vi "Controller Open Ethercat Variables.vi"(8 "error in (no error)":errorcluster, 11 "FOFB Configuration":T3={"FOFB Parameters"={"Network"={"FOFB Controller IP"="", "LNLS Control Network IP"="", "LNLS Control Network Power Supplies TCP Port"=0, "LNLS Control Network FOFB Configuration TCP Port"=0, "Data Server TCP Port"=0, "Monitoring Data TCP Port"=0, "Configuration GUI TCP Port"=0, "TCP Listening Timeout"=0}, "Fast Acquisition"={"Acquisition Period"=0, "Data Buffer Size"=0}, "Response Matrix Measurement"={"Step Amplitude"=0.0, "Time Between Steps"=0, "Step Duration"=0, "Number of Averages"=0}, "Correction Algorithm"={"Correction Period"=0, "Reference Orbit Path"=path "", "Response Matrix Path"=path "", "Correction Matrix Path"=path "", "Horizontal Correction Factor"=0.0, "Vertical Correction Factor"=0.0, "Beam Current FOFB Threshold"=0.0, "Decouple H-V"=FALSE}, "Acquisition Network"=[], "Actuation Network"=[]}, "Number of Acquisition Chassis"=0, "Number of Actuation Chassis"=0, "Number of BPM Readings"=0, "BPM Reading Names"=[], "Selected BPM Readings"=[0, 1, 2, 3, 4, 5, 6, 7, 8, 9, 10, 11, 12, 13, 14, 15, 16, 17, 18, 19, 20, 21, 22, 23, 24, 25, 26, 27, 28, 29, 30, 31, 32, 33, 34, 35, 36, 37, 38, 39, 40, 41, 42, 43, 44, 45, 46, 47, 48, 49], "Number of Correctors"=0, "Corrector Names"=[], "Selected Correctors"=[0, 1, 2, 3, 4, 5, 6, 7, 8, 9, 10, 11, 12, 13, 14, 15, 16, 17, 18, 19, 20, 21, 22, 23, 24, 25, 26, 27, 28, 29, 30, 31, 32, 33, 34, 35, 36, 37, 38, 39, 40, 41, 42, 43, 44, 45, 46, 47, 48, 49], "Reference Orbit"=[], "Response Matrix"=[], "Correction Matrix"=[], "Acquisition Chassis Names"=[], "Actuation Chassis Names"=[], "Acquisition Variables"=[], "Actuation Variables"=[], "PS Matrix Mapping"=[], "Inverse PS Matrix Mapping"=[], "Response Matrix Beam Energy (MeV)"=0.0, "PID Parameters"=[], "BPM Planes"=[], "Corrector Planes"=[], "RMM Step Factor"=[]}) -> (0 "error out":errorcluster, 2 "PS Variables":T1, 3 "BPM Variables":T2)   [LabVIEW 2011, in "Controller VIs.lvlib"]
doc: "Open references for all Acquisition and Actuation variables which are used to exchange data between the FOFB Controller and the Acquisition/Actuation chassis via the EtherCAT networks."
uses:
  Controller VIs.lvlib
  Types Definitions/Type FOFB Configuration.ctl
  Types Definitions/Type FOFB Parameters.ctl
  Types Definitions/Type Network Configuration.ctl
  Types Definitions/Type FA Configuration.ctl
  Types Definitions/Type Response Matrix Measurement Configuration.ctl
  Types Definitions/Type Correction Algorithm Configuration.ctl
  Types Definitions/Type Acquisition Network Configuration.ctl
  Types Definitions/Type Actuation Network Configuration.ctl
  Types Definitions/Type PID Parameters.ctl
  Types Definitions/Type BPM Variables.ctl
  Types Definitions/Type PS Variables.ctl
  Type Definitions.lvlib
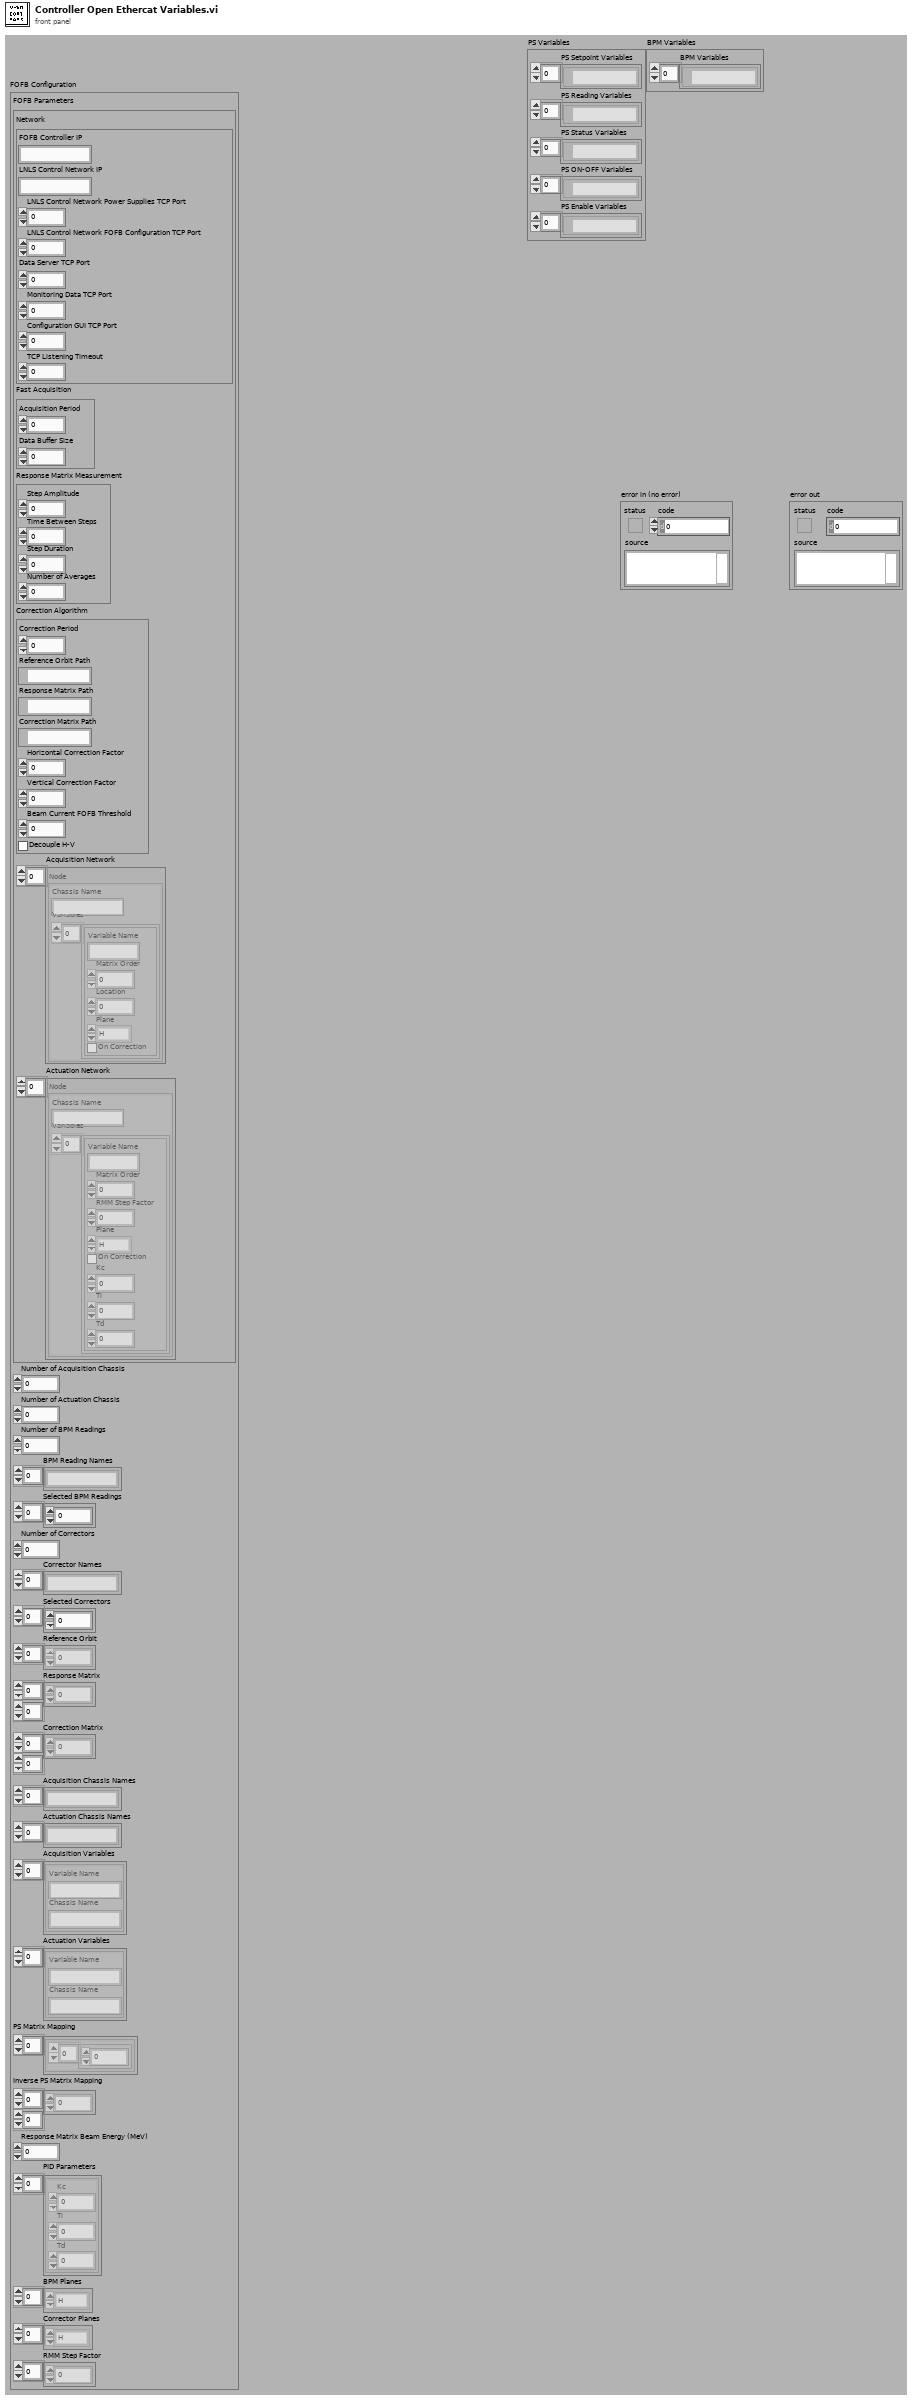
[diagram p1: front panel]
types:
  T1 = typedef "Type Definitions.lvlib/Type PS Variables.ctl" = cluster{"PS Setpoint Variables":refnum<k21>[], "PS Reading Variables":refnum<k21>[], "PS Status Variables":refnum<k21>[], "PS ON-OFF Variables":refnum<k21>[], "PS Enable Variables":refnum<k21>[]}
  T2 = typedef "Type Definitions.lvlib/Type BPM Variables.ctl" = cluster{"BPM Variables":refnum<k21>[]}
  T3 = typedef "Type Definitions.lvlib/Type FOFB Configuration.ctl" = cluster{"FOFB Parameters":T4, "Number of Acquisition Chassis":i32, "Number of Actuation Chassis":i32, "Number of BPM Readings":i32, "BPM Reading Names":string[], "Selected BPM Readings":u32[], "Number of Correctors":i32, "Corrector Names":string[], "Selected Correctors":u32[], "Reference Orbit":dbl[], "Response Matrix":dbl[][], "Correction Matrix":dbl[][], "Acquisition Chassis Names":string[], "Actuation Chassis Names":string[], "Acquisition Variables":cluster{"Variable Name":string, "Chassis Name":string}[], "Actuation Variables":cluster{"Variable Name":string, "Chassis Name":string}[], "PS Matrix Mapping":cluster{u32[]}[], "Inverse PS Matrix Mapping":u32[][], "Response Matrix Beam Energy (MeV)":dbl, "PID Parameters":T11[], "BPM Planes":enum8{"H", "V"}[], "Corrector Planes":enum8{"H", "V"}[], "RMM Step Factor":dbl[]}
  T4 = typedef "Type Definitions.lvlib/Type FOFB Parameters.ctl" = cluster{"Network":T5, "Fast Acquisition":T6, "Response Matrix Measurement":T7, "Correction Algorithm":T8, "Acquisition Network":T9, "Actuation Network":T10}
  T5 = typedef "Type Definitions.lvlib/Type Network Configuration.ctl" = cluster{"FOFB Controller IP":string, "LNLS Control Network IP":string, "LNLS Control Network Power Supplies TCP Port":u16, "LNLS Control Network FOFB Configuration TCP Port":u16, "Data Server TCP Port":u16, "Monitoring Data TCP Port":u16, "Configuration GUI TCP Port":u16, "TCP Listening Timeout":i32}
  T6 = typedef "Type Definitions.lvlib/Type FA Configuration.ctl" = cluster{"Acquisition Period":u32, "Data Buffer Size":u32}
  T7 = typedef "Type Definitions.lvlib/Type Response Matrix Measurement Configuration.ctl" = cluster{"Step Amplitude":dbl, "Time Between Steps":u32, "Step Duration":u32, "Number of Averages":u32}
  T8 = typedef "Type Definitions.lvlib/Type Correction Algorithm Configuration.ctl" = cluster{"Correction Period":u32, "Reference Orbit Path":path, "Response Matrix Path":path, "Correction Matrix Path":path, "Horizontal Correction Factor":dbl, "Vertical Correction Factor":dbl, "Beam Current FOFB Threshold":dbl, "Decouple H-V":bool}
  T9 = typedef "Type Definitions.lvlib/Type Acquisition Network Configuration.ctl" = cluster{"Chassis Name":string, "Variables":cluster{"Variable Name":string, "Matrix Order":u32, "Location":dbl, "Plane":enum8{"H", "V"}, "On Correction":bool}[]}[]
  T10 = typedef "Type Definitions.lvlib/Type Actuation Network Configuration.ctl" = cluster{"Chassis Name":string, "Variables":cluster{"Variable Name":string, "Matrix Order":u32, "RMM Step Factor":dbl, "Plane":enum8{"H", "V"}, "On Correction":bool, "Kc":dbl, "Ti":dbl, "Td":dbl}[]}[]
  T11 = typedef "Type Definitions.lvlib/Type PID Parameters.ctl" = cluster{"Kc":fxp<+/-,16,8>, "Ti":fxp<+/-,16,8>, "Td":fxp<+/-,16,8>}
  T12 = cluster{"Variable Name":string, "Chassis Name":string}[]
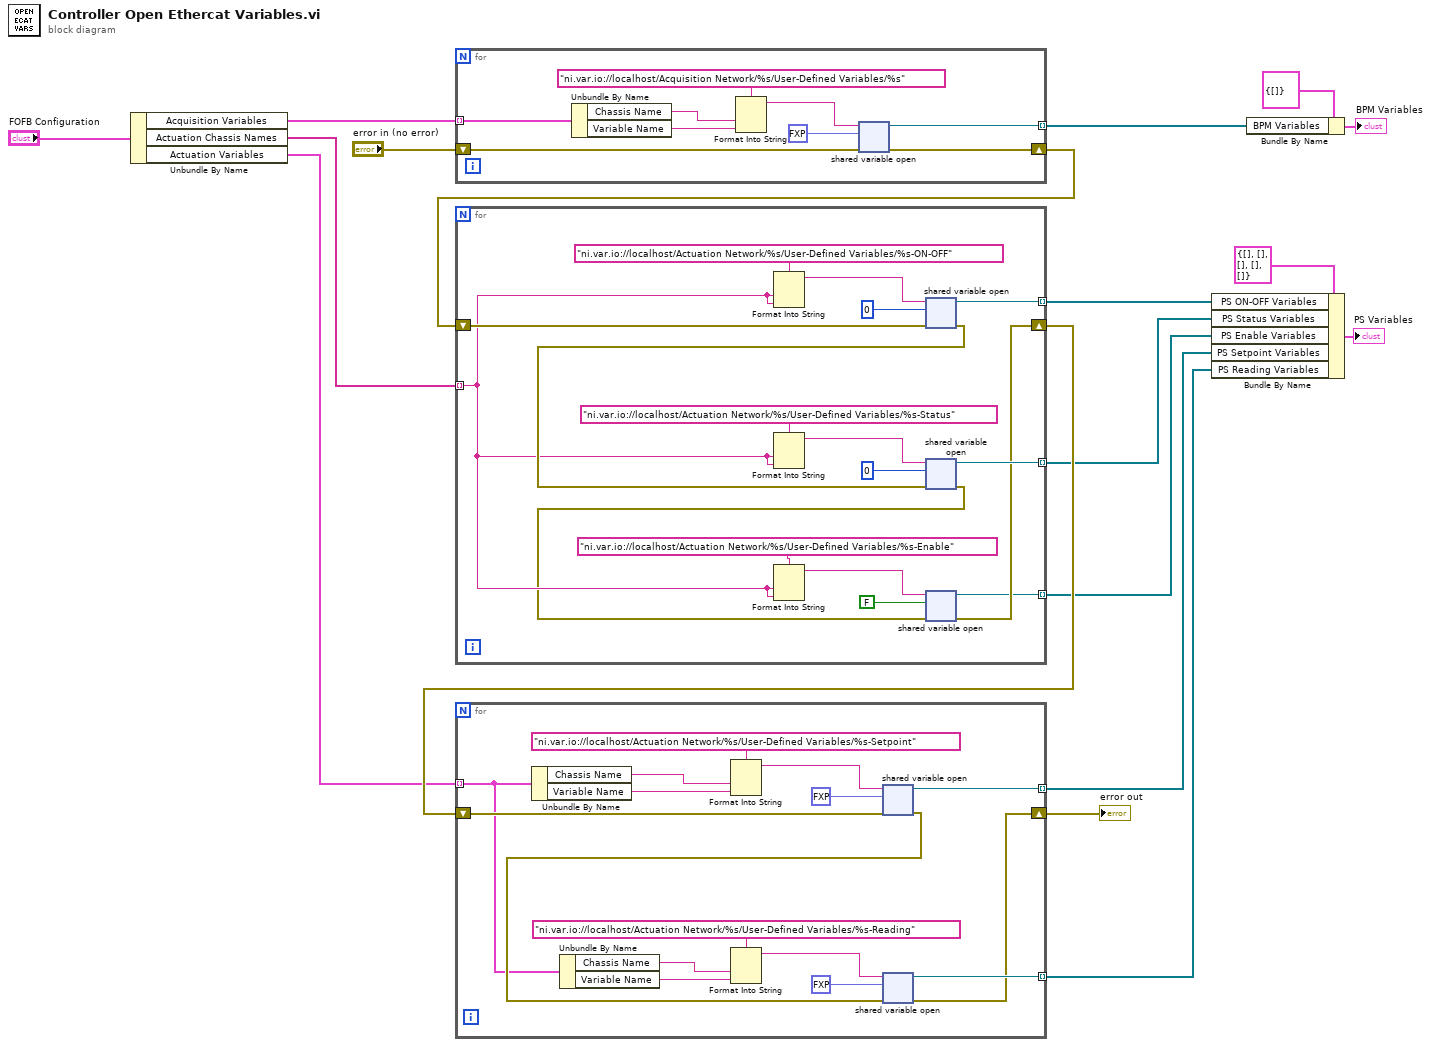
[diagram p0: block diagram]
diagram:
  n1 = Unbundle By Name("FOFB Configuration") -> ("Acquisition Variables"=w8:T12, "Actuation Chassis Names"=w7:string[], "Actuation Variables"=w6:T12)
  n2 = for {
    tunnel: w8 -> [w21] mode=indexing
    shift-right: [w26] -> w13
    shift-left: "error in (no error)" -> [w25]
    tunnel: [w24] -> w17 mode=indexing
    n3 = Unbundle By Name(w21) -> ("Chassis Name"=w20:string, "Variable Name"=w19:string)
    n4 = Format Into String(format string="ni.var.io://localhost/Acquisition Network/%s/User-Defined Variables/%s", w20, w19) -> (resulting string=w23:string)  [unwired: 2 in, 1 out]
    n5 = shared-variable-open(w23, w25, fxp<+/-,20,5> 0.0 ("BPM Data")) -> (w24:refnum<k21>, w26:errorcluster)  [unwired: 1 in]
  }
  n6 = for {
    shift-right: [w29] -> w12
    shift-left: w13 -> [w37]
    tunnel: w7 -> [w31] mode=indexing
    tunnel: [w36] -> w11 mode=indexing
    tunnel: [w35] -> w10 mode=indexing
    tunnel: [w28] -> w3 mode=indexing
    n7 = Format Into String(format string="ni.var.io://localhost/Actuation Network/%s/User-Defined Variables/%s-ON-OFF", w31, w31) -> (resulting string=w44:string)  [unwired: 2 in, 1 out]
    n8 = Format Into String(format string="ni.var.io://localhost/Actuation Network/%s/User-Defined Variables/%s-Status", w31, w31) -> (resulting string=w41:string)  [unwired: 2 in, 1 out]
    n9 = Format Into String(format string="ni.var.io://localhost/Actuation Network/%s/User-Defined Variables/%s-Enable", w31, w31) -> (resulting string=w33:string)  [unwired: 2 in, 1 out]
    n10 = shared-variable-open(w44, w37, u8 0) -> (w36:refnum<k21>, w40:errorcluster)  [unwired: 1 in]
    n11 = shared-variable-open(w41, w40, u8 0) -> (w35:refnum<k21>, w30:errorcluster)  [unwired: 1 in]
    n12 = shared-variable-open(w33, w30, FALSE) -> (w28:refnum<k21>, w29:errorcluster)  [unwired: 1 in]
  }
  n13 = for {
    shift-right: [w50] -> w15
    shift-left: w12 -> [w51]
    tunnel: w6 -> [w47] mode=indexing
    tunnel: [w55] -> w4 mode=indexing
    tunnel: [w54] -> w9 mode=indexing
    n14 = Unbundle By Name(w47) -> ("Chassis Name"=w49:string, "Variable Name"=w48:string)
    n15 = Unbundle By Name(w47) -> ("Chassis Name"=w45:string, "Variable Name"=w46:string)
    n16 = Format Into String(format string="ni.var.io://localhost/Actuation Network/%s/User-Defined Variables/%s-Setpoint", w49, w48) -> (resulting string=w60:string)  [unwired: 2 in, 1 out]
    n17 = Format Into String(format string="ni.var.io://localhost/Actuation Network/%s/User-Defined Variables/%s-Reading", w45, w46) -> (resulting string=w57:string)  [unwired: 2 in, 1 out]
    n18 = shared-variable-open(w60, w51, fxp<+/-,20,5> 0.0 ("PS Setpoint Data")) -> (w55:refnum<k21>, w56:errorcluster)  [unwired: 1 in]
    n19 = shared-variable-open(w57, w56, fxp<+/-,20,5> 0.0 ("PS Reading Data")) -> (w54:refnum<k21>, w50:errorcluster)  [unwired: 1 in]
  }
  "error out" <- w15
  n20 = Bundle By Name(cluster=T1 {"PS Setpoint Variables"=[], "PS Reading Variables"=[], "PS Status Variables"=[], "PS ON-OFF Variables"=[], "PS Enable Variables"=[]} ("output cluster"), "PS ON-OFF Variables"=w11, "PS Status Variables"=w10, "PS Enable Variables"=w3, "PS Setpoint Variables"=w4, "PS Reading Variables"=w9) -> (→"PS Variables":T1)
  n21 = Bundle By Name(cluster=T2 {"BPM Variables"=[]} ("output cluster"), "BPM Variables"=w17) -> (→"BPM Variables":T2)
